vi "Get JSON.vi"(11 "ConfigFromJSON in":refnum<class "Config from JSON.lvclass">) -> (2 "<JSON>":string, 3 "ConfigFromJSON out":refnum<class "Config from JSON.lvclass">)   [LabVIEW 2019, in "Configuration.lvlib" / "Config from JSON.lvclass"]
uses:
  Config from JSON.lvclass
  Config from JSON.lvclass/Config from JSON.ctl
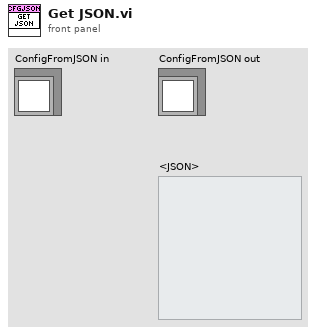
[diagram p1: front panel]
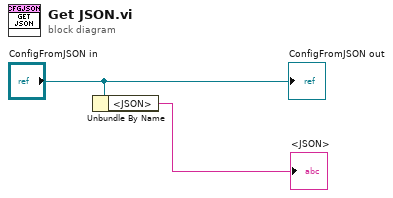
[diagram p0: block diagram]
diagram:
  n1 = Unbundle By Name("ConfigFromJSON in") -> ("<JSON>"=→"<JSON>":string)
  "ConfigFromJSON out" <- "ConfigFromJSON in"
